vi "forceToVoltage.vi"(8 "error in (no error)":errorcluster, 9 "Center Point":dbl[unit], 10 "Force":dbl[unit], 11 "ForceToPressureServoVoltage in":refnum<class "ForceToPressureServoVoltage.lvclass">) -> (0 "error out":errorcluster, 1 "Voltage 2":dbl[unit], 2 "Voltage 1":dbl[unit], 3 "ForceToPressureServoVoltage out":refnum<class "ForceToPressureServoVoltage.lvclass">)   [LabVIEW 2015, in "ForceToPressureServoVoltage.lvclass"]
uses:
  ForceToPressureServoVoltage.lvclass
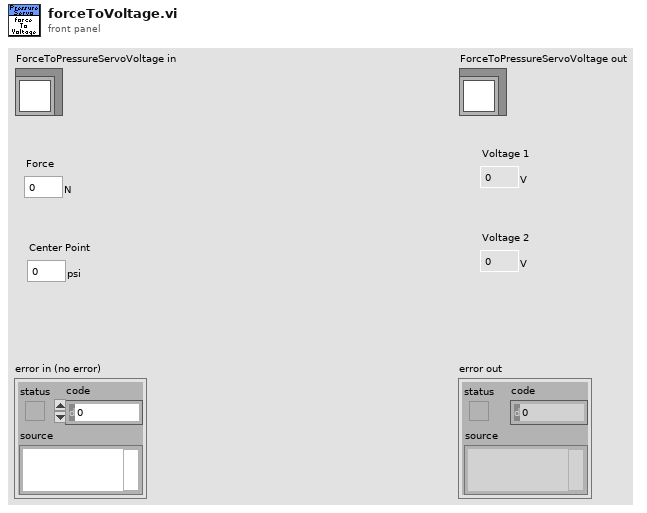
[diagram p1: front panel]
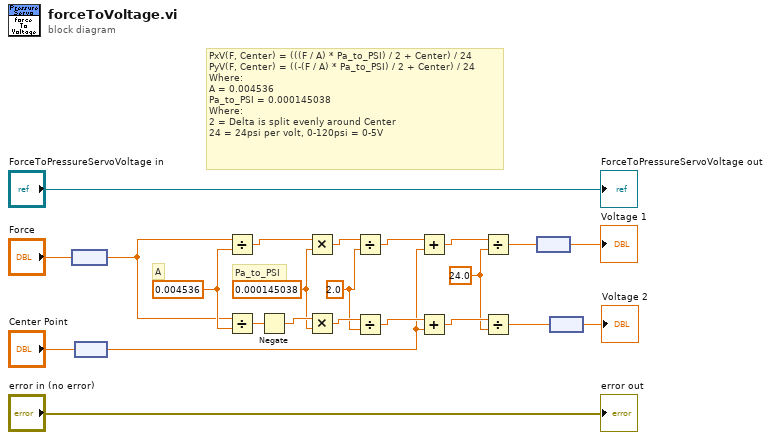
[diagram p0: block diagram]
diagram:
  w7 = 24.0 ("y")
  w16 = 2.0 ("y")
  w19 = 0.000145038
  w23 = 0.004536
  # "Pa_to_PSI"
  # "A"
  # "PxV(F, Center) = (((F / A) * Pa_to_PSI) / 2 + Center) / 24\nPyV(F, Center) = ((-(F / A) * Pa_to_PSI) / 2 + Center) / 24\nWhere:\nA = 0.004536\nPa_to_PSI = 0.000145038\nWhere:\n2 = Delta is split evenly around Center\n24 = 24psi per volt, 0-120psi = 0-5V"
  n1 = node("Force") -> (w12:dbl)
  n2 = node("Center Point") -> (w10:dbl)
  n3 = Divide(x=w12, y=w23) -> (x/y=w20:dbl)
  n4 = Divide(x=w12, y=w23) -> (x/y=w22:dbl)
  n5 = Negate(x=w22) -> (-x=w21:dbl)
  n6 = Multiply(x=w20, y=w19) -> (x*y=w18:dbl)
  n7 = Multiply(x=w21, y=w19) -> (x*y=w17:dbl)
  n8 = Divide(x=w18, y=w16) -> (x/y=w15:dbl)
  n9 = Divide(x=w17, y=w16) -> (x/y=w14:dbl)
  n10 = Add(x=w15, y=w10) -> (x+y=w9:dbl)
  n11 = Add(x=w14, y=w10) -> (x+y=w8:dbl)
  n12 = Divide(x=w9, y=w7) -> (x/y=w6:dbl)
  n13 = Divide(x=w8, y=w7) -> (x/y=w5:dbl)
  n14 = node(w6) -> (→"Voltage 1":dbl[unit])
  n15 = node(w5) -> (→"Voltage 2":dbl[unit])
  "error out" <- "error in (no error)"
  "ForceToPressureServoVoltage out" <- "ForceToPressureServoVoltage in"
